vi "PC Streaming Host with slow.vi"() -> ()   [LabVIEW 2012]
uses:
  <vilib>/userdefined/High Color/nirio_resource_hc.ctl
  hv cluster control.ctl
  Slow cluster control.ctl
  <vilib>/FPGAPlugInAG/PXI-7951R/niLvFpga_Open_PXI-7951R.vi
  <vilib>/rvi/interface/common/dynamic/niFpgaDynamicAddResources.vi
  <vilib>/Utility/error.llb/Error Cluster From Error Code.vi
  <vilib>/rvi/errors/niLvFpgaAdjustHostInterfaceError.vi
  <vilib>/FPGAPlugInAG/Dynamic/niLvFpga_Close_Dynamic.vi
  <vilib>/rvi/interface/nirviOpenFPGA/nirviOpenFPGA.xnode
  FPGA Bitfiles/ModuDAQ_FPGATarget_TopLevelFPGAw8LE_8T5P+CgHwo4.lvbitx
  <vilib>/rvi/interface/nirviReadWriteControl/nirviReadWriteControl.xnode
  <vilib>/rvi/interface/nirviMethod/nirviMethod.xnode
  <vilib>/rvi/interface/nirviCloseFPGA/nirviCloseFPGA.xnode
  <vilib>/ptbypt/NI_PtbyPt.lvlib
  <vilib>/rvi/interface/Simulation/niFpgaSimulationCallBeginRW.vi
  CAENHVs/CAEN/labview/CAENHVWrapper/CAENHVWrapper.lvlib
  NiFpgaLv.dll
  <vilib>/FPGAPlugInAG/Dynamic/niLvFpga_ReadFifo_Dynamic.vi
  <vilib>/rvi/errors/niLvFpgaMergeErrorWithErrorCode.vi
panel:
  out "fast loop stop":bool
  in  "Channel Cluster":T1={"det_type"=["", "", "", "", "", "", "", ""], "Serial numbers"=["", "", "", "", "", "", "", ""], "Sources"=["", "", "", "", "", "", "", ""], "Trigger level"=[4000, 4000, 4000, 4000, 4000, 4000, 4000, 4000], "Data Record On/Off"=[FALSE, FALSE, FALSE, FALSE, FALSE, FALSE, FALSE, FALSE, TRUE, FALSE, FALSE, FALSE, FALSE, FALSE, FALSE, TRUE], "Number of Channels"=8}
  in  "HV Cluster":T2={"HV Power On/Off"=[TRUE, TRUE], "Set Voltage(V)"=["0", "0", "0", "0", "0", "0", "0", "0"], "HV Tolerance (%)"=1.0, "Current(uA)"=[]}
  out "created path":path
  out "File name":string
  out "Total Data Chunks to Write":dbl
  in  "Tab Control":T3(tab)
  in  "Write mode":bool
  out "directory exists - please wait":u8(slide)
  out "directory ok":bool
  in  "Write Enable":bool
  in  "File Path":path=path "G:/"
  out "File Writing Progress (%)":dbl(slide) scale=0.0..100.0
  in  "Slow Control On":bool
  in  "Fast Data On":bool
  in  "Number of Files to Write":u32=1
  in  "IP Address of NIST Time Server":string(combo)="ntp1.nikhef.nl"
  in  "VISA resource name":refnum<visa-resource-name>="COM8"
  out "HV Power On/Off":bool[](array[boolean])=[TRUE, TRUE, TRUE, TRUE, TRUE, TRUE, TRUE, TRUE]
  in  "HV Tolerance (%)":dbl=1.0
  out "HV(V)":sgl[](array[numeric])
  in  "IP adress HV2":string="1_0_0"
  in  "IP adress HV1":string="0_0_0"
  out "error HV":errorcluster
  out "Set Voltage":string[](array[string])=["620", "510", "680", "700", "990", "670", "690", "760"]
  out "Current(uA)":sgl[](array[numeric])
  out "Current(uA) initial":sgl[](array[numeric])=[107.9, 102.05, 119.4, 122.0, 172.65, 116.8, 120.15, 132.35]
  in  "General Cluster":cluster{"Location":i16}={"Location"=1} {"Location" items=["Purdue", "NIKHEF", "Zurich", "???"]}
  in  "PXI address":T4="RIO0" caption="RIO Device"
  in  "det_type":string[](array[combo])=["NaI(Tl)", "NaI(Tl)", "NaI(Tl)", "NaI(Tl)", "NaI(Tl)", "NaI(Tl)", "NaI(Tl)", "NaI(Tl)"]
  in  "Serial numbers":string[](array[combo])=["SBJ593", "SBJ592", "SBJ590", "SBJ591", "SBJ588", "SBJ589", "SBJ586", "Other"]
  in  "Sources":string[](array[combo])=["Background", "Background", "Ti-44", "Ti-44", "Co-60", "Co-60", "Cs-137", "Cs-137"]
  in  "Trigger level":i16[](array[numeric])=[2000, 2000, 2000, 2000, 2000, 2000, 2000, 2000] caption="Trigger"
  in  "Data Record \nOn/Off":bool[](array[boolean])=[TRUE, TRUE, TRUE, TRUE, TRUE, TRUE, TRUE, TRUE]
  in  "Testpulse Cluster":T5={"Master Pulser On/Off"=FALSE, "Testpulse Turnaround Time (samples)"=14, "Pulse Separation (samples)"=0, "Pulse duration (samples)"=0}
  out "Samples per Data Chunk":u32
  in  "DAQ Info Cluster":T6={"Data Chunks per File"=1000, "Samples per Waveform"=95, "Pretrigger Samples"=15, "circular buffer length (samples)"=1000, "Waveforms per Data Chunk"=5000} {"Waveforms per Data Chunk" format="%.2p"}
  out "Average Throughput":dbl(graph)
  out "Loop Time":u32
  out "Inst. Throughput":dbl format="%#_6p"
  out "Elements in FIFO":u32(graph)
  out "FIFO Overflow":bool
  out "Current Chunk":u32
  out "Current File":i32
  out "Timeout Error":bool
  out "Elements Remaining":u32
  out "Waveform Graph":dynamicdata(graph)
  out "Channel number displayed":i16=-1
  in  "Arduino read \nrate (Hz)":dbl=1.0
  out "Slow time":u64
  out "data":dbl[](array[numeric])
  in  "XON Character":u8=17 format="%.0x"
  in  "XOFF Character":u8=19 format="%.0x"
  out "Slow Cluster":T7
  out "read buffer":string
  out "Bad sensor?":string
  in  "Max Slow Entries per File":i32=86400
  out "Current Slow File":i32
  out "Current Slow Entry":i32
  out "Sensor out of bounds":bool
  out "Temperature":dbl(graph)
  out "Pressure":dbl(graph)
  out "magnetic field y coordinate":dbl(graph)
  out "total magnetic field":dbl(graph)
  out "magnetic field z coordinate":dbl(graph)
  out "magnetic field x coordinate":dbl(graph)
  out "humidity":dbl(graph)
  out "XML String":string
  out "Slow XML":string
  out "error out FAST":errorcluster
  out "error out SLOW":errorcluster
  out "error out XML":errorcluster
  out "NIST Time":u64
  out "NIST Time Failed to Read":bool
  in  "Minutes to wait":u32=5 min=3
  out "UTC format":bool=TRUE
  out "FPGA Timestamp":u64
  out "Time stamp string":string
  out "Stopped":bool
  in  "stop":bool
  # "Channel 0"
  # "Channel 1"
  # "Channel 2"
  # "Channel 3"
  # "Channel 4"
  # "Channel 5"
  # "Channel 6"
  # "Channel 7"
  # "Write continuously"
  # "Write finite number of files"
  # "Program will stop when number of Files to Write is Complete OR if stop is pressed."
  # "These parameters are set by the set_shutdown_HV vi!"
  # "Channel 0"
  # "Channel 1"
  # "Channel 2"
  # "Channel 3"
  # "Channel 4"
  # "Channel 5"
  # "Channel 6"
  # "Channel 7"
  # "This is not a cluster"
  # "Channel 0"
  # "Channel 1"
  # "Channel 2"
  # "Channel 3"
  # "Channel 4"
  # "Channel 5"
  # "Channel 6"
  # "Channel 7"
  # "TODO: Make this look like the \"detectors\" tab"
  # "Waveform/Data Chunk information"
  # "To compare directly on a scope: Horizontal scale: 200 ns/div Vertical scale: ~100 mV/div If 15 pretriggers, delay = 700 ns"
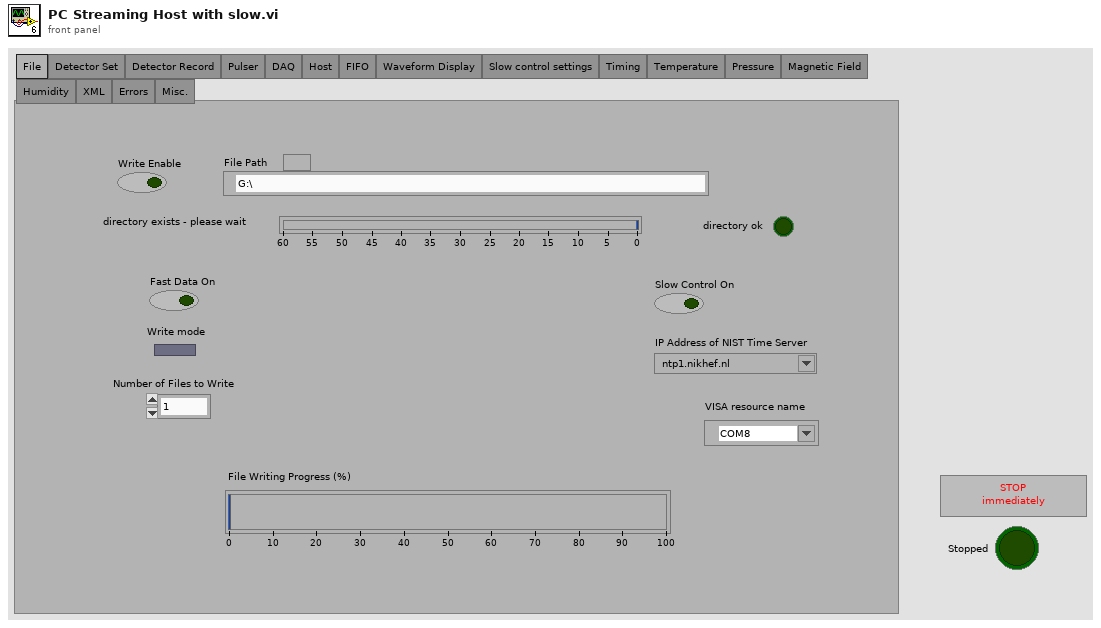
[diagram p1: front panel]
types:
  T1 = cluster{"det_type":string[], "Serial numbers":string[], "Sources":string[], "Trigger level":i16[], "Data Record On/Off":bool[], "Number of Channels":u8}
  T2 = typedef "hv cluster control.ctl" = cluster{"HV Power On/Off":bool[], "Set Voltage(V)":string[], "HV Tolerance (%)":dbl, "Current(uA)":dbl[]}
  T3 = enum32{"File", "Detector Set", "Detector Record", "Pulser", "DAQ", "Host", "FIFO", "Waveform Display", "Slow control settings", "Timing", "Temperature", "Pressure", "Magnetic Field", "Humidity", "XML", "Errors", "Misc."}
  T4 = typedef "nirio_resource_hc.ctl" = tag
  T5 = cluster{"Master Pulser On/Off":bool, "Testpulse Turnaround Time (samples)":u32, "Pulse Separation (samples)":u32, "Pulse duration (samples)":u32}
  T6 = cluster{"Data Chunks per File":u32, "Samples per Waveform":u32, "Pretrigger Samples":u32, "circular buffer length (samples)":u32, "Waveforms per Data Chunk":u32}
  T7 = typedef "Slow cluster control.ctl" = cluster{"Arduino \nParameters":dbl, "Total Number of \nSlow Parameters":i32, "UTC format?":bool, "Sensor Upper \nbounds":i32[], "Sensor Lower \nbounds":i32[], "Descriptions":string[], "datanames":string[]}
  T8 = enum16{"open", "replace", "create", "open or create", "replace or create", "replace or create with confirmation"}
  T9 = enum16{"big-endian, network order", "native, host order", "little-endian"}
  T10 = cluster{"Arduino Parameters":dbl, "Total Number of Slow Parameters":i32, "UTC format?":bool, "Sensor Upper bounds":i32[], "Sensor Lower bounds":i32[], "Descriptions":string[], "datanames":string[]}
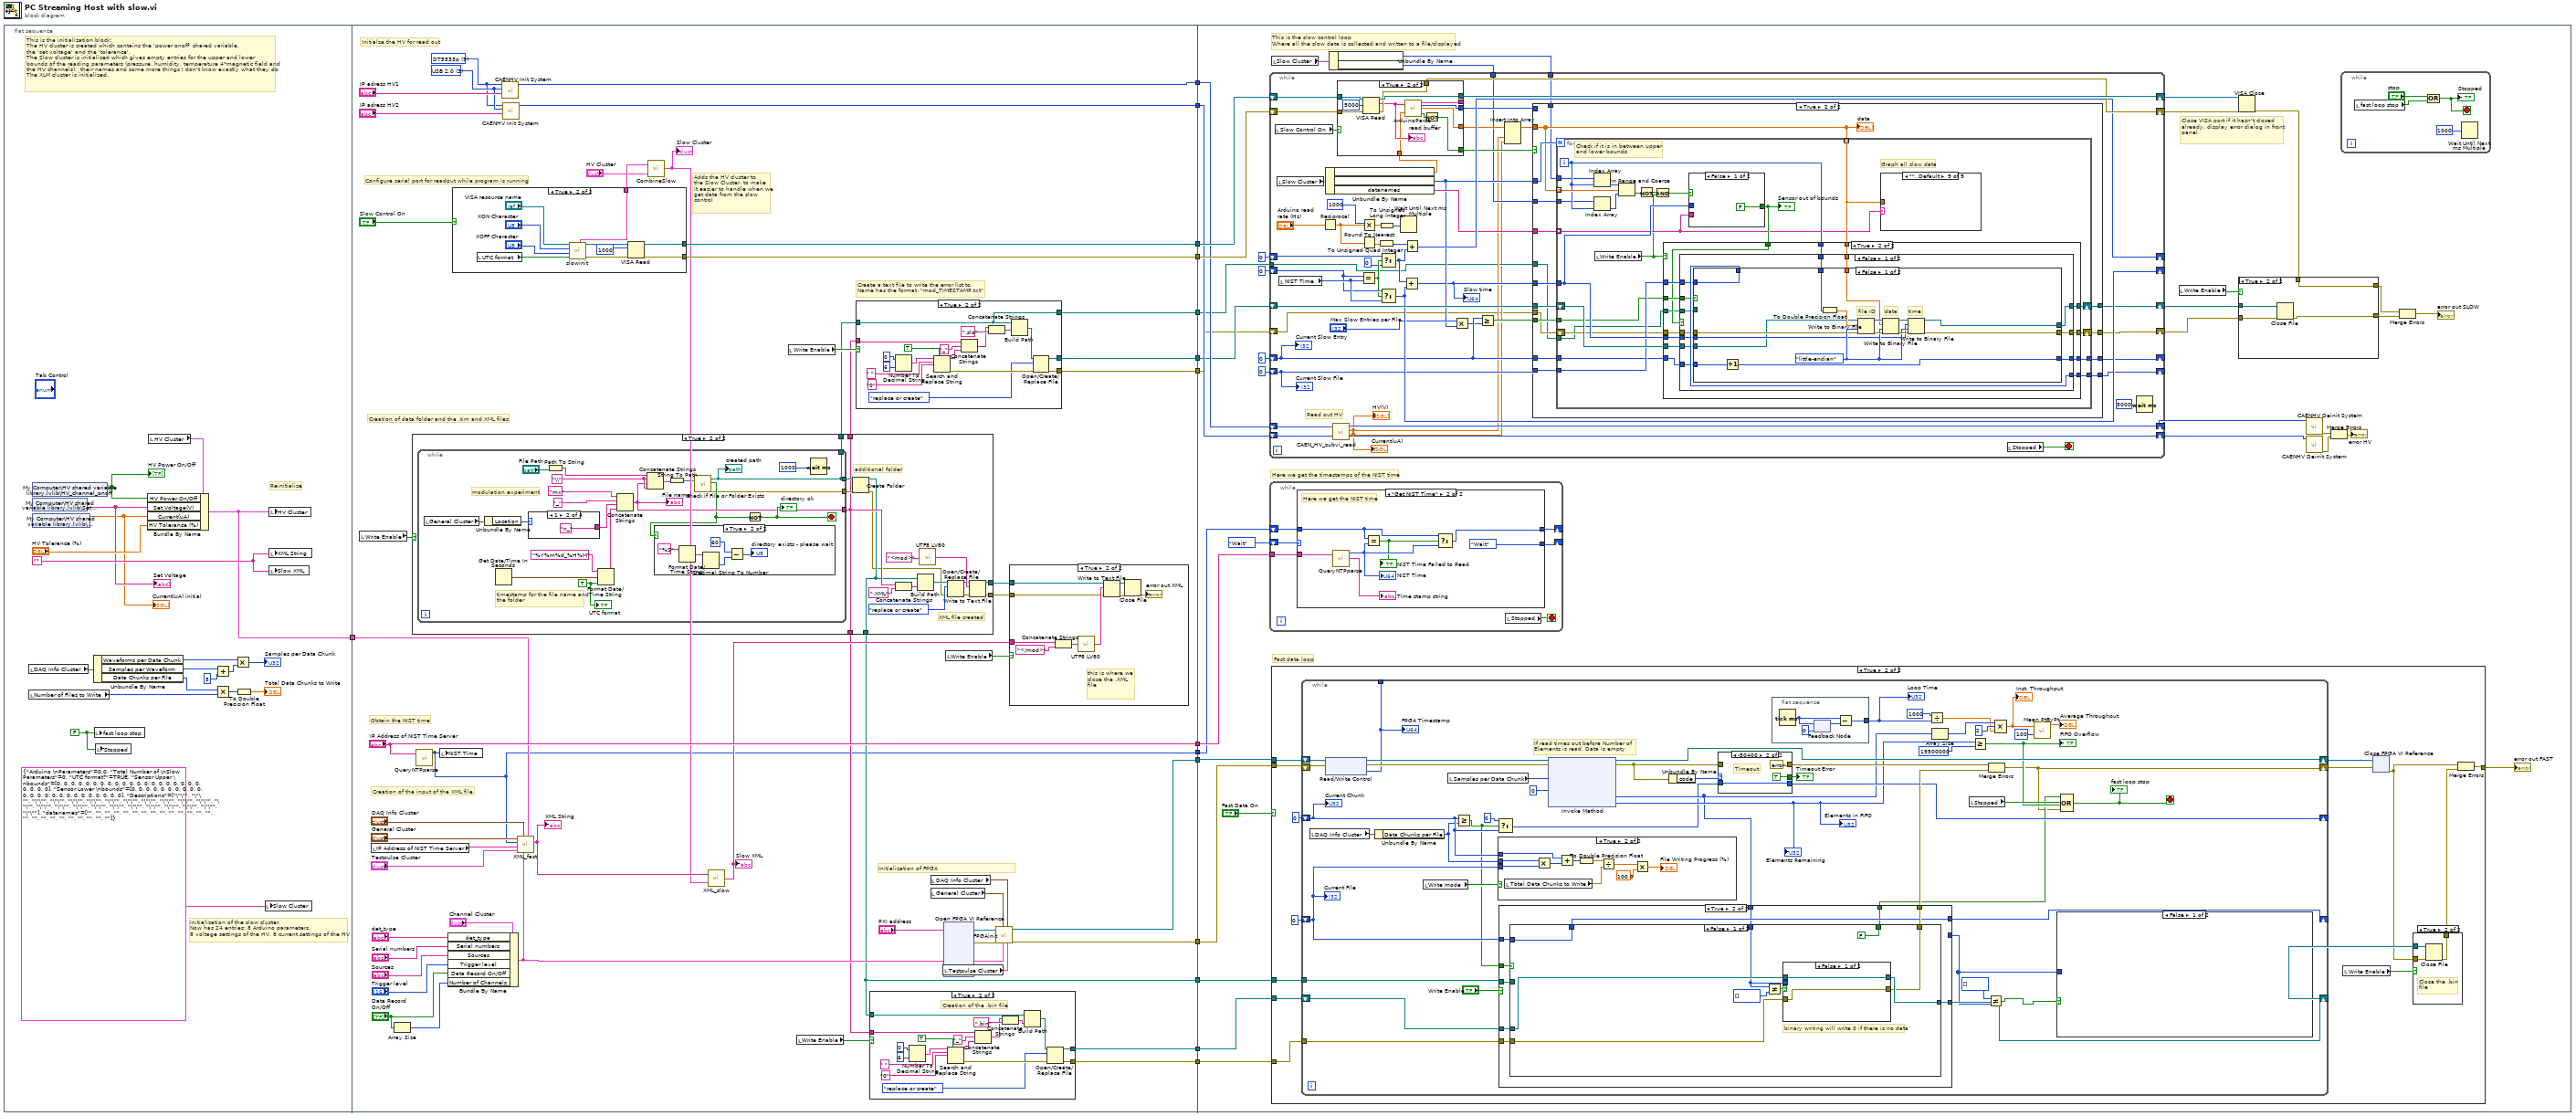
[diagram p0: block diagram]
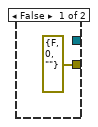
[diagram p2: hidden frame]
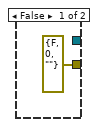
[diagram p3: hidden frame]
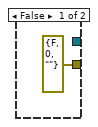
[diagram p6: hidden frame]
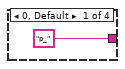
[diagram p7: hidden frame]
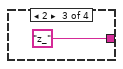
[diagram p8: hidden frame]
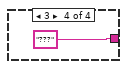
[diagram p9: hidden frame]
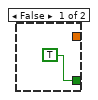
[diagram p11: hidden frame]
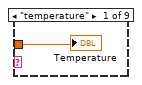
[diagram p13: hidden frame]
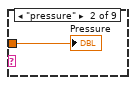
[diagram p14: hidden frame]
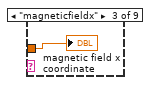
[diagram p15: hidden frame]
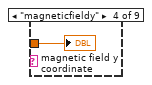
[diagram p16: hidden frame]
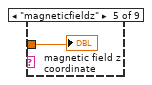
[diagram p17: hidden frame]
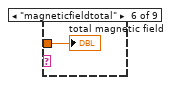
[diagram p18: hidden frame]
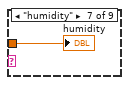
[diagram p19: hidden frame]
diagram:
  n1 = flat-sequence {
    tunnel: [w22] -> w4
    tunnel: ["IP Address of NIST Time Server"] -> w15
    tunnel: [w63] -> w14
    tunnel: [w62] -> w13
    tunnel: [w58] -> w12
    tunnel: [w57] -> w11
    tunnel: [w56] -> w10
    tunnel: [w47] -> w9
    tunnel: [w46] -> w8
    tunnel: [w45] -> w7
    tunnel: [w41] -> w6
    tunnel: [w40] -> w5
    tunnel: w4 -> [w39]
    tunnel: [w38] -> w3
    tunnel: [w37] -> w2
    tunnel: [w36] -> w1
    tunnel: w15 -> [w220]
    tunnel: w14 -> [w212]
    tunnel: w13 -> [w211]
    tunnel: w12 -> [w208]
    tunnel: w11 -> [w210]
    tunnel: w10 -> [w209]
    tunnel: w9 -> [w207]
    tunnel: w8 -> [w206]
    tunnel: w7 -> [w205]
    tunnel: w6 -> [w204]
    tunnel: w5 -> [w203]
    tunnel: w3 -> [w202]
    tunnel: w2 -> [w197]
    tunnel: w1 -> [w194]
    frame #0 {
      w20 = FALSE ("fast loop stop")
      w34 = ""
      # "Initialization of the slow cluster.\nNow has 24 entries: 8 Arduino parameters, \n8 voltage settings of the HV, 8 current settings of the HV"
      # "This is the initialization block!\nThe HV cluster is created which contains the 'power onoff' shared variable, \nthe 'set voltage' and the 'tolerance'.\nThe Slow cluster is initialized which gives empty entries for the upper and lower\nbounds of the reading parameters (pressure, humidity, temperature 4*magnetic field and\nthe HV channels),  their names and some more things I don't know exactly what they do\nThe XLM cluster is initialized."
      # "Reinitialize"
      n2 = local read "DAQ Info Cluster"() -> (w32:T6)
      n3 = local read "Number of Files to Write"() -> (w27:u32)
      n4 = shared-variable "My Computer\\HV shared variable library.lvlib\\HV_channel_onoff"() -> (w18:bool[])  [unwired: 1 in, 1 out]
      "HV Power On/Off" <- w18
      n5 = shared-variable "My Computer\\HV shared variable library.lvlib\\Set Voltage"() -> (w17:string[])  [unwired: 1 in, 1 out]
      "Set Voltage" <- w17
      n6 = shared-variable "My Computer\\HV shared variable library.lvlib\\Current(uA)"() -> (w16:dbl[])  [unwired: 1 in, 1 out]
      "Current(uA) initial" <- w16
      n7 = Unbundle By Name(w32) -> ("Waveforms per Data Chunk"=w24:u32, "Samples per Waveform"=w25:u32, "Data Chunks per File"=w26:u32)
      n8 = local write "fast loop stop"(w20) -> ()
      n9 = local write "Stopped"(w20) -> ()
      n10 = local read "HV Cluster"() -> (w33:T2)
      n11 = Bundle By Name(cluster=w33, "HV Power On/Off"=w18, "Set Voltage(V)"=w17, "Current(uA)"=w16, "HV Tolerance (%)"="HV Tolerance (%)") -> (w22:T2)
      n12 = Add(x=w25, y=u32 5) -> (x+y=w29:u32)
      n13 = Multiply(x=w26, y=w27) -> (x*y=w31:u32)
      n14 = Multiply(x=w24, y=w29) -> (x*y=→"Samples per Data Chunk":u32)
      n15 = To Double Precision Float(number=w31) -> (double precision float=→"Total Data Chunks to Write":dbl)
      n16 = local write "Slow Cluster"(T7 {"Arduino \nParameters"=0.0, "Total Number of \nSlow Parameters"=0, "UTC format?"=TRUE, "Sensor Upper \nbounds"=[0, 0, 0, 0, 0, 0, 0, 0, 0, 0, 0, 0, 0, 0, 0, 0, 0, 0, 0, 0, 0, 0, 0, 0], "Sensor Lower \nbounds"=[0, 0, 0, 0, 0, 0, 0, 0, 0, 0, 0, 0, 0, 0, 0, 0, 0, 0, 0, 0, 0, 0, 0, 0], "Descriptions"=["\"\"", "\"\"", "\"\"", "\"\"", "\"\"", "\"\"", "\"\"", "\"\"", "\"\"", "\"\"", "\"\"", "\"\"", "\"\"", "\"\"", "\"\"", "\"\"", "\"\"", "\"\"", "\"\"", "\"\"", "\"\"", "\"\"", "\"\"", "\"\""], "datanames"=["", "", "", "", "", "", "", "", "", "", "", "", "", "", "", "", "", "", "", "", "", "", "", ""]} ("Slow Cluster 2")) -> ()
      n17 = local write "HV Cluster"(w22) -> ()
      n18 = local write "XML String"(w34) -> ()
      n19 = local write "Slow XML"(w34) -> ()
    }
    frame #1 {
      w65 = 3 items=["TCP/IP"=0, "HS CAENET"=2, "USB 2.0"=3, "CONET Optical Link"=4, "USB VCP"=5] ("LinkType")
      w64 = u32 9 items=["SY1527", "SY2527", "SY4527", "SY5527", "N568", "V65XX", "N1470", "V8100", "", "DT5533p"] ("system")
      # "Obtain the NIST time"
      # "Adds the HV cluster to\nthe Slow Cluster, to make\nit easier to handle when we\nget data from the slow\ncontrol"
      # "Initialization of FPGA"
      # "Initialze the HV for read out"
      # "Create a text file to write the error list to.  \nName has the format: \"mod_TIMESTAMP.txt\""
      # "Creation of the input of the XML file"
      # "Configure serial port for readout while program is running"
      # "Creation of data folder and the .tim and XML files"
      n20 = local read "Write Enable"() -> (w86:bool)
      n21 = local read "IP Address of NIST Time Server"() -> (w77:string)
      n22 = Array Size(array="Data Record \nOn/Off") -> (size(s)=w75:i32)
      n23 = case shown="True" w86 {
        tunnel: [_ w158] -> w59
        tunnel: [_ w150] -> w61
        tunnel: [_ w148] -> w48
        tunnel: [_ w148] -> w42
        tunnel: [_ w147] -> w41
        tunnel: [errorcluster {"status"=FALSE, "code"=0, "source"=""} ("error out") w145] -> w35
        frame False {
        }
        frame True {
          # "XML file created"
          # "additional folder"
          n24 = while {
            tunnel: [w161] -> w159
            tunnel: [w163] -> w160
            tunnel: [w163] -> w158
            tunnel: [w168] -> w148
            stop <- w173 stop-if-true
            w169 = "\\" ("string")
            w176 = TRUE ("UTC format")
            # "modulation experiment"
            # "timestamp for the file name and the folder"
            n25 = local read "General Cluster"() -> (w166:cluster{"Location":i16})
            n26 = Unbundle By Name(w166) -> ("Location"=w165:i16)
            n27 = Get Date/Time In Seconds() -> (seconds since 1Jan1904=w177:timestamp)
            n28 = case shown="1" w165 {
              tunnel: ["p_" ("string") "n_" ("string") "z_" ("string") "???"] -> w167
              frame 0, Default {
              }
              frame 1 {
              }
              frame 2 {
              }
              frame 3 {
              }
            }
            n29 = Path To String(path="File Path") -> (string=w179:string)
            n30 = Format Date/Time String(time format string (%c)="%Y%m%d_%H%M", seconds (now)=w177, UTC format=w176) -> (date/time string=w170:string)
            n31 = Concatenate Strings("mx" ("string"), "_" ("string"), w167, w170) -> (w168:string)
            "File name" <- w168
            n32 = Concatenate Strings(w179, w169, w168, w169) -> (w180:string)
            n33 = String To Path(string=w180) -> (path=w164:path)
            n34 = call <vilib>:"Check if File or Folder Exists.vi"("path"=w164) -> ("error out"=w161:errorcluster, "file or folder exists?"=w162:bool, "dup path"=w163:path)  [unwired: 8 in]
            "created path" <- w163
            n35 = case shown="True" w162 {
              frame False {
              }
              frame True {
                n36 = Format Date/Time String(time format string (%c)="%S") -> (date/time string=w188:string)  [unwired: 2 in]
                n37 = Decimal String To Number(string=w188) -> (number=w186:i32)  [unwired: 2 in, 1 out]
                n38 = Subtract(x=60, y=w186) -> (x-y=→"directory exists - please wait":i32)
              }
            }
            n39 = Not(x=w162) -> (.not. x?=w173:bool)
            "directory ok" <- w173
            n40 = Wait (ms)(milliseconds to wait=1000) -> ()  [unwired: 1 out]
            "UTC format" <- w176
          }
          n41 = Create Folder(path (use dialog)=w160, error in=w159) -> (created path=w147:path, error out=w146:errorcluster)  [unwired: 1 in, 1 out]
          n42 = Concatenate Strings(w148, ".XML" ("substring (\"\")")) -> (w154:string)
          n43 = Build Path(base path=w147, name or relative path=w154) -> (appended path=w153:path)
          n44 = call "UTF8 LV80.vi"("text"="<mod>") -> ("utf-8 text out"=w157:string)
          n45 = Open/Create/Replace File(file path (use dialog)=w153, error in=w146, operation (0:open)=T8."replace or create") -> (refnum out=w156:refnum<file>, error out=w155:errorcluster)  [unwired: 3 in, 1 out]
          n46 = Write to Text File(file (use dialog)=w156, text=w157, error in=w155) -> (refnum out=w150:refnum<file>, error out=w145:errorcluster)  [unwired: 1 in, 1 out]
        }
      }
      n47 = call "QueryNTPparse.vi"("IP Address of NIST Server"="IP Address of NIST Time Server") -> ("NTP Time (server time)"=w38:u64)  [unwired: 1 in, 2 out]
      n48 = local write "NIST Time"(w38) -> ()
      n49 = Bundle By Name(cluster="Channel Cluster", "det_type"="det_type", "Serial numbers"="Serial numbers", "Sources"="Sources", "Trigger level"="Trigger level", "Data Record On/Off"="Data Record \nOn/Off", "Number of Channels"=w75) -> (w44:T1)
      n50 = case shown="True" "Slow Control On" {
        tunnel: [_ w143] -> w63
        tunnel: [_ w142] -> w62
        tunnel: [_ w134] -> w85
        frame False {
        }
        frame True {
          n51 = local read "UTC format"() -> (w137:bool)
          n52 = call "slowinit.vi"("UTC format"=w137, "XOFF Character"="XOFF Character", "XON Character"="XON Character", "VISA resource name"="VISA resource name") -> ("error IO"=w135:errorcluster, "VISA resource name out"=w136:refnum<visa-resource-name>, "Slow Cluster"=w134:T10)  [unwired: 5 in]
          n53 = VISA Read(VISA resource name=w136, byte count=u32 1000, error in (no error)=w135) -> (VISA resource name out=w143:refnum<visa-resource-name>, error out=w142:errorcluster)  [unwired: 2 out]
        }
      }
      n54 = call "CAENHV Init System.vi"("Arg"="IP adress HV1", "LinkType"=w65, "system"=w64) -> ("handle"=w57:i32)  [unwired: 7 in, 1 out]
      n55 = call "CAENHV Init System.vi"("Arg"="IP adress HV2", "LinkType"=w65, "system"=w64) -> ("handle"=w56:i32)  [unwired: 7 in, 1 out]
      n56 = call "XML_fast.vi"("HV Cluster"=w39, "Channel \nCluster"=w44, "DAQ Info Cluster"="DAQ Info Cluster", "Testpulse \nCluster"="Testpulse Cluster", "IP Address of NIST Time Server"=w77, "NIST Time"=w38, "General Cluster"="General Cluster") -> ("XML String"=w80:string)  [unwired: 4 in]
      "XML String" <- w80
      n57 = call "CombineSlow.vi"("HV Cluster"="HV Cluster", "Slow Cluster in"=w85) -> ("Slow Cluster"=w43:T7)
      "Slow Cluster" <- w43
      n58 = call "XML_slow.vi"("Slow Cluster"=w43, "Input String"=w80) -> ("Output String"=w81:string)
      "Slow XML" <- w81
      n59 = local read "Write Enable"() -> (w60:bool)
      n60 = local read "Write Enable"() -> (w49:bool)
      n61 = case shown="True" w60 {
        tunnel: [_ w117] -> w58
        tunnel: w48 -> [_ w109]
        tunnel: w59 -> [_ w108]
        tunnel: [_ w108] -> w40
        tunnel: [errorcluster {"status"=FALSE, "code"=0, "source"=""} ("error out") w107] -> w37
        frame False {
        }
        frame True {
          n62 = Number To Decimal String(number=0, width (-)=i16 6) -> (decimal integer string=w124:string)
          n63 = Search and Replace String(replace all?=TRUE ("replace all? (F)"), input string=w124, search string=" ", replace string="0" ("replace string (\"\")")) -> (result string=w114:string, error out=w119:errorcluster)  [unwired: 4 in, 2 out]
          n64 = Concatenate Strings(w109, "_" ("string"), w114) -> (w112:string)
          n65 = Concatenate Strings(w112, ".slo" ("substring (\"\")")) -> (w116:string)
          n66 = Build Path(base path=w108, name or relative path=w116) -> (appended path=w120:path)
          n67 = Open/Create/Replace File(file path (use dialog)=w120, error in=w119, operation (0:open)=T8."replace or create") -> (refnum out=w117:refnum<file>, error out=w107:errorcluster)  [unwired: 3 in, 1 out]
        }
      }
      n68 = case shown="True" w49 {
        tunnel: [_ w98] -> w47
        tunnel: w42 -> [_ w90]
        tunnel: w41 -> [_ w89]
        tunnel: [errorcluster {"status"=FALSE, "code"=0, "source"=""} ("error out") w88] -> w36
        frame False {
        }
        frame True {
          # "Creation of the .bin file"
          n69 = Number To Decimal String(number=0, width (-)=i16 6) -> (decimal integer string=w105:string)
          n70 = Search and Replace String(replace all?=TRUE ("replace all? (F)"), input string=w105, search string=" ", replace string="0" ("replace string (\"\")")) -> (result string=w95:string, error out=w100:errorcluster)  [unwired: 4 in, 2 out]
          n71 = Concatenate Strings(w90, "_" ("string"), w95) -> (w93:string)
          n72 = Concatenate Strings(w93, ".bin" ("substring (\"\")")) -> (w97:string)
          n73 = Build Path(base path=w89, name or relative path=w97) -> (appended path=w101:path)
          n74 = Open/Create/Replace File(file path (use dialog)=w101, error in=w100, operation (0:open)=T8."replace or create") -> (refnum out=w98:refnum<file>, error out=w88:errorcluster)  [unwired: 3 in, 1 out]
        }
      }
      n75 = local read "DAQ Info Cluster"() -> (w53:T6)
      n76 = local read "General Cluster"() -> (w52:cluster{"Location":i16})
      n77 = local read "Testpulse Cluster"() -> (w51:T5)
      n78 = xnode "Open FPGA VI Reference"("resource name"="PXI address") -> ("FPGA VI Reference Out"=w55:refnum<k20>, "error out"=w54:errorcluster)  [unwired: 1 in]
      n79 = local read "Write Enable"() -> (w68:bool)
      n80 = call "FPGAinit.vi"("Testpulse Cluster"=w51, "DAQ Info Cluster"=w53, "Channel Cluster"=w44, "General Cluster"=w52, "error in"=w54, "FPGA VI Reference In"=w55) -> ("error out"=w45:errorcluster, "FPGA VI Reference Out"=w46:refnum<k20>)  [unwired: 4 in]
      n81 = case shown="True" w68 {
        tunnel: w61 -> [_ w133]
        tunnel: w81 -> [_ w128]
        tunnel: w35 -> [_ w127]
        frame False {
        }
        frame True {
          # "this is where we close the .XML file"
          n82 = Concatenate Strings(w128, "</mod>" ("string")) -> (w129:string)
          n83 = call "UTF8 LV80.vi"("text"=w129) -> ("utf-8 text out"=w132:string)
          n84 = Write to Text File(file (use dialog)=w133, text=w132, error in=w127) -> (refnum out=w131:refnum<file>, error out=w126:errorcluster)  [unwired: 1 in, 1 out]
          n85 = Close File(refnum=w131, error in=w126) -> (error out=→"error out XML":errorcluster)  [unwired: 1 out]
        }
      }
    }
    frame #2 {
      # "This is the slow control loop\nWhere all the slow data is collected and written to a file/displayed"
      # "Fast data loop"
      # "Close VISA port if it hasn't closed already, display error dialog in front panel"
      # "Here we get the timestamps of the NIST time"
      n86 = while {
        shift-right: [w617] -> _
        shift-left: enum16{"Wait", "Get NIST Time", "Write"}."Wait" -> [w618]
        shift-right: [w616] -> _
        shift-left: w202 -> [w615]
        tunnel: w220 -> [w614]
        stop <- w613 stop-if-true
        n87 = case shown="\"Get NIST Time\"" w618 {
          tunnel: [w621 enum16{"Wait", "Get NIST Time", "Write"}."Wait"] -> w617
          tunnel: [w620 w637] -> w616
          tunnel: w615 -> [w620 w634]
          tunnel: w614 -> [_ w633]
          frame "Wait", Default {
            # "First we wait 'minutes to wait' and proceed with Getting the NIST time\nthis is necessary to see a  drift, if it is there, between the PFGA and NIST time"
            n88 = while {
              tunnel: [enum16{"Wait", "Get NIST Time", "Write"}."Get NIST Time"] -> w621
              tunnel: "Minutes to wait" -> [w623]
              i -> [w626]
              stop <- w627 stop-if-true
              n89 = local read "Stopped"() -> (w625:bool)
              n90 = Multiply(x=60, y=w623) -> (x*y=w622:u32)
              n91 = Wait Until Next ms Multiple(millisecond multiple=u32 1000 ("y")) -> ()  [unwired: 1 out]
              n92 = Greater Or Equal?(x=w626, y=w622) -> (x >= y?=w628:bool)
              n93 = Or(x=w628, y=w625) -> (x .or. y?=w627:bool)
            }
          }
          frame "Get NIST Time" {
            # "Here we get the NIST time"
            n94 = call "QueryNTPparse.vi"("IP Address of NIST Server"=w633) -> ("NTP Time (server time)"=w636:u64, "Time stamp string"=→"Time stamp string":string)  [unwired: 1 in, 1 out]
            "NIST Time" <- w636
            n95 = Equal?(x=w634, y=w636) -> (x = y?=w635:bool)
            "NIST Time Failed to Read" <- w635
            n96 = Select(t=w634, s=w635, f=w636) -> (s? t:f=w637:u64)
          }
        }
        n97 = local read "Stopped"() -> (w613:bool)
      }
      n98 = local read "Slow Cluster"() -> (w224:T7)
      n99 = case shown="True" "Fast Data On" {
        tunnel: w207 -> [_ w450]
        tunnel: w206 -> [_ w449]
        tunnel: w205 -> [w440 w448]
        tunnel: w204 -> [_ w447]
        tunnel: [w440 w442] -> w195
        tunnel: w194 -> [_ w441]
        frame False {
        }
        frame True {
          n100 = while {
            shift-right: [w462] -> w445
            shift-left: w448 -> [w481]
            shift-right: [w488] -> _
            shift-left: u32 0 -> [w485]
            shift-right: [w473] -> _
            shift-left: 0 ("number") -> [w474]
            shift-right: [w489] -> w452
            shift-left: w450 -> [w490]
            tunnel: [w478] -> _
            tunnel: w447 -> [w466]
            shift-right: [w505] -> w446
            shift-left: w449 -> [w468]
            tunnel: w441 -> [w461]
            stop <- w475 stop-if-true
            # "If read times out before Number of Elements is read, Data is empty"
            n101 = local read "DAQ Info Cluster"() -> (w470:T6)
            n102 = xnode "Read/Write Control"("FPGA VI Reference In"=w468, "error in"=w481) -> ("FPGA VI Reference Out"=w480:refnum<k20>, "error out"=w479:errorcluster, "Timestamp"=w478:u64)
            "FPGA Timestamp" <- w478
            n103 = Unbundle By Name(w470) -> ("Data Chunks per File"=w469:u32)
            n104 = local read "Write mode"() -> (w482:bool)
            n105 = local read "Samples per Data Chunk"() -> (w467:u32)
            n106 = Greater Or Equal?(x=w485, y=w469) -> (x >= y?=w463:bool)
            n107 = Select(t=u32 0, s=w463, f=w485) -> (s? t:f=w465:u32)
            n108 = case shown="True" w482 {
              tunnel: w474 -> [_ w524]
              tunnel: w485 -> [_ w522]
              tunnel: w469 -> [_ w515]
              frame False {
              }
              frame True {
                n109 = local read "Total Data Chunks to Write"() -> (w519:dbl)
                n110 = Multiply(x=w515, y=w524) -> (x*y=w523:u32)
                n111 = Add(x=w522, y=w523) -> (x+y=w521:u32)
                n112 = To Double Precision Float(number=w521) -> (double precision float=w520:dbl)
                n113 = Divide(x=w520, y=w519) -> (x/y=w517:dbl)
                n114 = Multiply(x=w517, y=100.0) -> (x*y=→"File Writing Progress (%)":dbl)
              }
            }
            n115 = xnode "Invoke Method"("FPGA VI Reference In"=w480, "error in"=w479, "Number of Elements"=w467, "Timeout (ms)"=0) -> ("FPGA VI Reference Out"=w505:refnum<k20>, "error out"=w502:errorcluster, "Data"=w483:i16[], "Elements Remaining"=w484:u32)
            "Elements in FIFO" <- w484
            "Elements Remaining" <- w484
            n116 = case shown="True" "Write Enable" {
              tunnel: w483 -> [w532 w534]
              tunnel: [w532 _] -> w472
              tunnel: w463 -> [_ w543]
              tunnel: [w529 w542] -> w491
              tunnel: [w533 w541] -> w489
              tunnel: w490 -> [w533 w540]
              tunnel: w474 -> [w531 w539]
              tunnel: [w531 w538] -> w473
              tunnel: [FALSE w537] -> w464
              tunnel: w466 -> [_ w536]
              tunnel: w461 -> [w529 w535]
              frame False {
              }
              frame True {
                n117 = case shown="False" w543 {
                  tunnel: w534 -> [w548 w576]
                  tunnel: [w547 w578] -> w542
                  tunnel: w540 -> [w552 w591]
                  tunnel: [w551 w584] -> w541
                  tunnel: w539 -> [w546 w564]
                  tunnel: [w546 w563] -> w538
                  tunnel: [FALSE w562] -> w537
                  tunnel: w536 -> [_ w565]
                  tunnel: w535 -> [w544 w561]
                  frame False {
                    # "binary writing will write 0 if there is no data"
                    n118 = Not Equal?(x=w548, y=i16[] []) -> (x != y?=w549:bool)
                    n119 = case shown="False" w549 {
                      tunnel: w552 -> [w554 w560]
                      tunnel: [w554 w559] -> w551
                      tunnel: [w553 w558] -> w547
                      tunnel: w548 -> [_ w556]
                      tunnel: w544 -> [w553 w555]
                      frame False {
                      }
                      frame True {
                        n120 = Write to Binary File(file (use dialog)=w560, data=w556, error in=w555, 9:T9."little-endian" ("byte order (0:big-endian, network order)")) -> (refnum out=w559:refnum<file>, error out=w558:errorcluster)  [unwired: 2 in, 1 out]
                      }
                    }
                  }
                  frame True {
                    # "little-endian is windows and linux way of writing and reading binary not the standard in labview !?!"
                    # "opening the new ones"
                    # "closing files"
                    n121 = Increment(x=w564) -> (x+1=w563:i32)
                    n122 = Number To Decimal String(number=w563, width (-)=i16 6) -> (decimal integer string=w593:string)
                    n123 = Close File(refnum=w591, error in=w561) -> (error out=w590:errorcluster)  [unwired: 1 out]
                    n124 = local read "File name"() -> (w572:string)
                    n125 = Search and Replace String(replace all?=TRUE ("replace all? (F)"), input string=w593, search string=" ", replace string="0" ("replace string (\"\")"), error in=w590) -> (result string=w583:string, error out=w589:errorcluster)  [unwired: 3 in, 2 out]
                    n126 = Concatenate Strings(w572, "_" ("string"), w583) -> (w579:string)
                    n127 = local read "Samples per Data Chunk"() -> (w571:u32)
                    n128 = Concatenate Strings(w579, ".bin" ("substring (\"\")")) -> (w581:string)
                    n129 = Equal?(x="Write mode", y=TRUE) -> (x = y?=w570:bool)
                    n130 = Equal?(x="Number of Files to Write", y=w563) -> (x = y?=w569:bool)
                    n131 = And(x=w569, y=w570) -> (x .and. y?=w562:bool)
                    n132 = Build Path(base path=w565, name or relative path=w581) -> (appended path=w588:path)
                    n133 = Open/Create/Replace File(file path (use dialog)=w588, error in=w589, operation (0:open)=T8."replace or create") -> (refnum out=w585:refnum<file>, error out=w586:errorcluster)  [unwired: 3 in, 1 out]
                    n134 = Array Size(array=w576) -> (size(s)=w575:i32)
                    n135 = Equal?(x=w575, y=w571) -> (x = y?=w574:bool)
                    n136 = Not Equal?(x=w576, y=i16[] []) -> (x != y?=w577:bool)
                    n137 = And(x=w577, y=w574) -> (x .and. y?=w573:bool)
                    n138 = case shown="True" w573 {
                      tunnel: w586 -> [w598 w605]
                      tunnel: w585 -> [w599 w604]
                      tunnel: [w599 w603] -> w584
                      tunnel: [w598 w602] -> w578
                      tunnel: w576 -> [_ w601]
                      frame False {
                      }
                      frame True {
                        n139 = Write to Binary File(file (use dialog)=w604, data=w601, error in=w605, 9:T9."little-endian" ("byte order (0:big-endian, network order)")) -> (refnum out=w603:refnum<file>, error out=w602:errorcluster)  [unwired: 2 in, 1 out]
                      }
                    }
                  }
                }
              }
            }
            n140 = Unbundle By Name(w502) -> ("code"=w503:i32)
            n141 = case shown="-50400" w503 {
              tunnel: [w609 errorcluster {"status"=FALSE, "code"=0, "source"=""} ("error constant")] -> w492
              tunnel: w502 -> [w609 _]
              tunnel: w465 -> [w608 w611]
              tunnel: [w607 w611] -> w488
              tunnel: [FALSE TRUE] -> w459
              frame 0, Default {
                n142 = Increment(x=w608) -> (x+1=w607:u32)
              }
              frame -50400 {
                # "Timeout"
              }
            }
            "Timeout Error" <- w459
            n143 = flat-sequence {
              tunnel: [w528] -> w496
              frame #0 {
                n144 = Tick Count (ms)() -> (millisecond timer value=w527:u32)
                n145 = feedback #1(u32 0 ("millisecond timer value")) -> (w526:u32)
                n146 = feedback-in #1(w527) -> ()
                n147 = Subtract(x=w527, y=w526) -> (x-y=w528:u32)
              }
            }
            n148 = Divide(x=u32 1000, y=w496) -> (x/y=w498:dbl)
            n149 = Array Size(array=w483) -> (size(s)=w501:i32)
            n150 = local read "Stopped"() -> (w477:bool)
            n151 = Greater Or Equal?(x=w484, y=u32 19500000) -> (x >= y?=w476:bool)
            "FIFO Overflow" <- w476
            n152 = Not Equal?(x=i16[] [], y=w472) -> (x != y?=w460:bool)
            n153 = Merge Errors(w492, w491) -> (w462:errorcluster)
            n154 = Compound Arithmetic op=MULTIPLY(w501, 2 ("y"), w498) -> (w495:dbl)
            "Inst. Throughput" <- w495
            n155 = call <vilib>:"Mean PtByPt.vi"("x"=w495, "sample length"=100) -> ("mean"=→"Average Throughput":dbl)  [unwired: 2 in, 1 out]
            n156 = case shown="False" w460 {
              tunnel: w472 -> [_ w514]
              frame False {
              }
              frame True {
                # "If Fast data isn't empty and\nno data is written to a file\nthe waveform will be plotted"
                n157 = local read "Channel Cluster"() -> (w512:T1)
                n158 = local read "General Cluster"() -> (w510:cluster{"Location":i16})
                n159 = local read "DAQ Info Cluster"() -> (w508:T6)
                n160 = Unbundle By Name(w512) -> ("Trigger level"=w511:i16[])
                n161 = Unbundle By Name(w510) -> ("Location"=w509:i16)
                n162 = Unbundle By Name(w508) -> ("Samples per Waveform"=w507:u32)
                n163 = call "displaydaqwave.vi"("Samples per Waveform"=w507, "Location"=w509, "Trigger level"=w511, "Waveform from DAQ"=w514) -> ("Waveform Graph"=→"Waveform Graph":dynamicdata, "Channel number displayed"=→"Channel number displayed":i16)  [unwired: 6 in]
              }
            }
            n164 = Compound Arithmetic op=OR(w464, w477, w476, w462) -> (w475:bool)
            "fast loop stop" <- w475
            "Loop Time" <- w496
            "Current Chunk" <- w485
            "Current File" <- w474
          }
          n165 = local read "Write Enable"() -> (w454:bool)
          n166 = xnode "Close FPGA VI Reference"("FPGA VI Reference In"=w446, "error in"=w445) -> ("error out"=w444:errorcluster)
          n167 = case shown="True" w454 {
            tunnel: w444 -> [w455 w457]
            tunnel: w452 -> [_ w458]
            tunnel: [w455 w456] -> w443
            frame False {
            }
            frame True {
              # "Close the .bin\nfile"
              n168 = Close File(refnum=w458, error in=w457) -> (error out=w456:errorcluster)  [unwired: 1 out]
            }
          }
          n169 = Merge Errors(w444, w443) -> (w442:errorcluster)
        }
      }
      "error out FAST" <- w195
      n170 = Unbundle By Name(w224) -> ("Sensor Upper \nbounds"=w214:i32[], "Sensor Lower \nbounds"=w213:i32[])
      n171 = while {
        shift-right: [w270] -> _
        shift-left: u64 0 -> [w274]
        shift-right: [w267] -> _
        shift-left: u64 0 -> [w272]
        shift-right: [w253] -> w219
        shift-left: w208 -> [w276]
        shift-right: [w249] -> _
        shift-left: 0 -> [w250]
        shift-right: [w248] -> _
        shift-left: 0 -> [w252]
        tunnel: w214 -> [w242]
        tunnel: w213 -> [w241]
        tunnel: w203 -> [w232]
        shift-right: [w278] -> w216
        shift-left: w212 -> [w240]
        shift-right: [w277] -> w215
        shift-left: w211 -> [w239]
        shift-right: [w236] -> w218
        shift-left: w210 -> [w238]
        shift-right: [w234] -> w217
        shift-left: w209 -> [w237]
        shift-right: [w229] -> w196
        shift-left: w197 -> [w230]
        stop <- w233 stop-if-true
        # "Read out HV"
        n172 = local read "Slow Control On"() -> (w256:bool)
        n173 = local read "Slow Cluster"() -> (w261:T7)
        n174 = local read "NIST Time"() -> (w275:u64)
        n175 = Reciprocal(x="Arduino read \nrate (Hz)") -> (1/x=w264:dbl)
        n176 = Unbundle By Name(w261) -> ("Arduino \nParameters"=w257:dbl, "Total Number of \nSlow Parameters"=w246:i32, "datanames"=w254:string[])
        n177 = call "CAEN_HV_subvi_read.vi"("handle HV1"=w238, "handle HV2"=w237) -> ("handle HV1 out"=w236:i32, "HV"=w235:sgl[], "Current"=w231:sgl[], "handle HV2 out"=w234:i32)  [unwired: 1 in, 1 out]
        "HV(V)" <- w235
        "Current(uA)" <- w231
        n178 = case shown="True" w256 {
          tunnel: [_ w290] -> w278
          tunnel: [_ w289] -> w277
          tunnel: [_ w287] -> w260
          tunnel: [_ w286] -> _
          tunnel: [TRUE w282] -> w255
          tunnel: [_ w284] -> w259
          tunnel: w257 -> [_ w283]
          tunnel: w240 -> [_ w281]
          tunnel: w239 -> [_ w280]
          frame False {
          }
          frame True {
            n179 = VISA Read(VISA resource name=w281, byte count=u32 5000, error in (no error)=w280) -> (VISA resource name out=w290:refnum<visa-resource-name>, read buffer=w288:string, error out=w289:errorcluster)  [unwired: 1 out]
            "read buffer" <- w288
            n180 = call "ArduinoParse.vi"("read buffer"=w288, "Expected Arduino Parameters"=w283) -> ("Number Arduino Parameters"=w287:i32, "Arduino Data Names"=w286:string[], "Arduino Data"=w284:dbl[], "Arduino Read Failed?"=w285:bool)
            n181 = Not(x=w285) -> (.not. x?=w282:bool)
          }
        }
        n182 = Equal?(x=w274, y=w275) -> (x = y?=w273:bool)
        n183 = Multiply(x=u32 1000 ("millisecond multiple"), y=w264) -> (x*y=w266:dbl)
        n184 = Round To Nearest(number=w264) -> (nearest integer value=w263:dbl)
        n185 = To Unsigned Quad Integer(1:w263) -> (0:w262:u64)
        n186 = To Unsigned Long Integer(number=w266) -> (unsigned 32bit integer=w265:u32)
        n187 = Select(t=w272, s=w273, f=0) -> (s? t:f=w268:u64)
        n188 = Select(t=w274, s=w273, f=w275) -> (s? t:f=w270:u64)
        n189 = Wait Until Next ms Multiple(millisecond multiple=w265) -> ()  [unwired: 1 out]
        n190 = Add(x=w268, y=w270) -> (x+y=w243:u64)
        "Slow time" <- w243
        n191 = Add(x=w262, y=w268) -> (x+y=w267:u64)
        n192 = Multiply(x="Max Slow Entries per File", y=w246) -> (x*y=w245:i32)
        n193 = Greater Or Equal?(x=w250, y=w245) -> (x >= y?=w251:bool)
        n194 = Insert Into Array(array=w259, new element #1=w235, new element #2=w231) -> (w258:dbl[])  [unwired: 1 in]
        n195 = case shown="True" w255 {
          tunnel: w276 -> [w295 w311]
          tunnel: w243 -> [_ w310]
          tunnel: [w295 w307] -> w253
          tunnel: w260 -> [_ _]
          tunnel: w258 -> [_ w301]
          tunnel: w254 -> [_ w309]
          tunnel: w246 -> [_ w308]
          tunnel: w252 -> [w293 w306]
          tunnel: w251 -> [_ w305]
          tunnel: w250 -> [w294 w304]
          tunnel: [w294 w303] -> w249
          tunnel: [w293 w302] -> w248
          tunnel: w242 -> [_ w300]
          tunnel: w241 -> [_ w299]
          tunnel: w232 -> [_ w296]
          tunnel: w230 -> [w292 w298]
          tunnel: [w292 w297] -> w229
          frame False {
          }
          frame True {
            n196 = for {
              N: w308 -> [_]
              tunnel: w310 -> [w332]
              tunnel: w301 -> [w334] mode=indexing
              tunnel: w309 -> [w320] mode=indexing
              tunnel: w301 -> [w321] mode=indexing
              tunnel: w306 -> [w329]
              tunnel: w305 -> [w327]
              tunnel: w304 -> [w326]
              tunnel: [w325] -> w303
              tunnel: [w324] -> w302
              shift-right: [w330] -> w307
              shift-left: w311 -> [w331]
              tunnel: w300 -> [w319]
              tunnel: w299 -> [w318]
              shift-right: [w315] -> w297
              shift-left: w298 -> [w314]
              tunnel: w296 -> [w313]
              i -> [w328]
              # "Check if it is in between upper \nand lower bounds"
              # "Graph all slow data"
              n197 = Index Array(array=w319, index=w328) -> (element=w316:i32)
              n198 = Index Array(array=w318, index=w328) -> (element=w317:i32)
              n199 = local read "Write Enable"() -> (w312:bool)
              n200 = In Range and Coerce(upper limit=w316, x=w334, lower limit=w317) -> (In Range?=w323:bool)  [unwired: 1 out]
              n201 = Not(x=w323) -> (.not. x?=w335:bool)
              n202 = And(x=w335, y=w312) -> (x .and. y?=w333:bool)
              n203 = case shown="False" w333 {
                tunnel: w320 -> [_ w428]
                tunnel: w332 -> [_ _]
                tunnel: [FALSE ("Sensor out of bounds") TRUE ("Sensor out of bounds")] -> w322
                frame False {
                }
                frame True {
                  "Bad sensor?" <- w428
                }
              }
              "Sensor out of bounds" <- w322
              n204 = case shown="True" w312 {
                tunnel: [w344 w360] -> w324
                tunnel: w321 -> [_ w359]
                tunnel: w332 -> [_ w358]
                tunnel: w331 -> [w346 w357]
                tunnel: [w346 w356] -> w330
                tunnel: w329 -> [w344 w355]
                tunnel: w328 -> [_ w354]
                tunnel: w327 -> [_ w353]
                tunnel: w326 -> [w345 w352]
                tunnel: [w345 w351] -> w325
                tunnel: w322 -> [_ w350]
                tunnel: w313 -> [_ w349]
                tunnel: [w343 w348] -> w315
                tunnel: w314 -> [w343 w347]
                frame False {
                }
                frame True {
                  n205 = case shown="False" w350 {
                    tunnel: [w373 w425] -> w360
                    tunnel: w359 -> [w372 _]
                    tunnel: w358 -> [w371 _]
                    tunnel: w357 -> [w370 w424]
                    tunnel: [w369 w424] -> w356
                    tunnel: w355 -> [w368 w425]
                    tunnel: w354 -> [w367 _]
                    tunnel: w353 -> [w366 _]
                    tunnel: w352 -> [w365 w426]
                    tunnel: [w364 w426] -> w351
                    tunnel: w349 -> [w363 _]
                    tunnel: [w362 w423] -> w348
                    tunnel: w347 -> [w361 w423]
                    frame False {
                      n206 = case shown="False" w366 {
                        tunnel: [w381 w395] -> w373
                        tunnel: w372 -> [w383 w403]
                        tunnel: w371 -> [w382 w402]
                        tunnel: w370 -> [w375 w401]
                        tunnel: [w377 w399] -> w369
                        tunnel: w368 -> [w381 w398]
                        tunnel: w367 -> [w380 w397]
                        tunnel: w365 -> [w379 _]
                        tunnel: [w378 0] -> w364
                        tunnel: w363 -> [_ w393]
                        tunnel: [w374 w391] -> w362
                        tunnel: w361 -> [w376 w392]
                        frame False {
                          w384 = T9."little-endian" ("byte order (0:big-endian, network order)")
                          # "time"
                          # "data"
                          # "file ID"
                          n207 = Increment(x=w379) -> (x+1=w378:i32)
                          n208 = To Double Precision Float(number=w380) -> (double precision float=w385:dbl)
                          n209 = Write to Binary File(file (use dialog)=w375, data=w385, error in=w376, 9:w384) -> (refnum out=w388:refnum<file>, error out=w389:errorcluster)  [unwired: 2 in, 1 out]
                          n210 = Write to Binary File(file (use dialog)=w388, data=w383, error in=w389, 9:w384) -> (refnum out=w387:refnum<file>, error out=w386:errorcluster)  [unwired: 2 in, 1 out]
                          n211 = Write to Binary File(file (use dialog)=w387, data=w382, error in=w386, 9:w384) -> (refnum out=w377:refnum<file>, error out=w374:errorcluster)  [unwired: 2 in, 1 out]
                        }
                        frame True {
                          w404 = T9."little-endian" ("byte order (0:big-endian, network order)")
                          w394 = TRUE ("replace all? (F)")
                          # "time"
                          # "data"
                          # "file ID"
                          # "opening the new ones"
                          # "closing files"
                          n212 = Increment(x=w398) -> (x+1=w395:i32)
                          n213 = Number To Decimal String(number=w395, width (-)=i16 6) -> (decimal integer string=w419:string)
                          n214 = Close File(refnum=w401, error in=w392) -> (error out=w417:errorcluster)  [unwired: 1 out]
                          n215 = local read "File name"() -> (w410:string)
                          n216 = Search and Replace String(replace all?=w394, case sensitive?=w394, input string=w419, search string=" ", replace string="0" ("replace string (\"\")"), error in=w417) -> (result string=w414:string, error out=w416:errorcluster)  [unwired: 2 in, 2 out]
                          n217 = Concatenate Strings(w410, "_" ("string"), w414) -> (w411:string)
                          n218 = Concatenate Strings(w411, ".slo" ("substring (\"\")")) -> (w412:string)
                          n219 = Build Path(base path=w393, name or relative path=w412) -> (appended path=w390:path)
                          n220 = Open/Create/Replace File(file path (use dialog)=w390, error in=w416, operation (0:open)=T8."replace or create") -> (refnum out=w400:refnum<file>)  [unwired: 3 in, 2 out]
                          n221 = To Double Precision Float(number=w397) -> (double precision float=w405:dbl)
                          n222 = Write to Binary File(file (use dialog)=w400, data=w405, 9:w404) -> (refnum out=w408:refnum<file>, error out=w409:errorcluster)  [unwired: 3 in, 1 out]
                          n223 = Write to Binary File(file (use dialog)=w408, data=w403, error in=w409, 9:w404) -> (refnum out=w407:refnum<file>, error out=w406:errorcluster)  [unwired: 2 in, 1 out]
                          n224 = Write to Binary File(file (use dialog)=w407, data=w402, error in=w406, 9:w404) -> (refnum out=w399:refnum<file>, error out=w391:errorcluster)  [unwired: 2 in, 1 out]
                        }
                      }
                    }
                    frame True {
                    }
                  }
                }
              }
              n225 = case shown="\"\", Default" w320 {
                tunnel: w321 -> [w336 w337 w338 w339 w340 w341 w342 _ _]
                frame "temperature" {
                  "Temperature" <- w336
                }
                frame "pressure" {
                  "Pressure" <- w337
                }
                frame "magneticfieldx" {
                  "magnetic field x coordinate" <- w338
                }
                frame "magneticfieldy" {
                  "magnetic field y coordinate" <- w339
                }
                frame "magneticfieldz" {
                  "magnetic field z coordinate" <- w340
                }
                frame "magneticfieldtotal" {
                  "total magnetic field" <- w341
                }
                frame "humidity" {
                  "humidity" <- w342
                }
                frame "seconds" {
                }
                frame "", Default {
                }
              }
            }
            "data" <- w301
          }
        }
        n226 = local read "Stopped"() -> (w233:bool)
        n227 = Wait (ms)(milliseconds to wait=u32 5000) -> ()  [unwired: 1 out]
        "Current Slow Entry" <- w250
        "Current Slow File" <- w252
      }
      n228 = local read "Write Enable"() -> (w225:bool)
      n229 = VISA Close(VISA resource name=w216, error in (no error)=w215) -> (error out=w193:errorcluster)
      n230 = case shown="True" w225 {
        tunnel: w219 -> [_ w435]
        tunnel: w196 -> [w430 w434]
        tunnel: w193 -> [w431 w432]
        tunnel: [w430 w433] -> w192
        tunnel: [w431 w432] -> w191
        frame False {
        }
        frame True {
          n231 = Close File(refnum=w435, error in=w434) -> (error out=w433:errorcluster)  [unwired: 1 out]
        }
      }
      n232 = call "CAENHV Deinit System.vi"("handle"=w218) -> ("error out"=w223:errorcluster)  [unwired: 10 in]
      n233 = call "CAENHV Deinit System.vi"("handle"=w217) -> ("error out"=w222:errorcluster)  [unwired: 10 in]
      n234 = Merge Errors(w223, w222) -> (→"error HV":errorcluster)
      n235 = while {
        stop <- w437 stop-if-true
        n236 = local read "fast loop stop"() -> (w436:bool)
        n237 = Compound Arithmetic op=OR("stop", w436) -> (w437:bool)
        "Stopped" <- w437
        n238 = Wait Until Next ms Multiple(millisecond multiple=u32 1000 ("y")) -> ()  [unwired: 1 out]
      }
      n239 = Merge Errors(w191, w192) -> (→"error out SLOW":errorcluster)
    }
  }
